vi "LED_Perform Measurements.vi"(8 "error in":errorcluster, 9 "Voltage Values":dbl[](array[numeric]), 11 "Measurement Config_In":T1={"Load channel name"="", "Load out"="", "Source out"="", "Source channel name"="", "Source sequence name"="", "Voltage values"=[], "Voltage values-CV"=[], "Voltage values-LED"=[], "Output Resistance-LED"=[], "Source terminal name"="", "Measure terminal name"="", "Load Voltage-out"=[], "Load Current - out"=[], "Source Voltage-out"=[], "Source Current - out"=[], "LED Mode Start?"=FALSE, "LED Mode Completed?"=FALSE, "CalculateRd"=0.0, "Set LED Current Limit?"=FALSE, "OutputVoltageOffset"=0.0, "measurement results"={"Status"="Empty", "Source voltages"=[0.0], "Load voltages"=[0.0], "Source current"=[0.0], "Load current"=[0.0]}}) -> (0 "error Out":errorcluster, 1 "Measurement Data":T3, 3 "Measurement Config_Out":T1={"Load channel name"="", "Load out"="", "Source out"="", "Source channel name"="", "Source sequence name"="", "Voltage values"=[], "Voltage values-CV"=[], "Voltage values-LED"=[], "Output Resistance-LED"=[], "Source terminal name"="", "Measure terminal name"="", "Load Voltage-out"=[], "Load Current - out"=[], "Source Voltage-out"=[], "Source Current - out"=[], "LED Mode Start?"=FALSE, "LED Mode Completed?"=FALSE, "CalculateRd"=0.0, "Set LED Current Limit?"=FALSE, "OutputVoltageOffset"=0.0, "measurement results"={"Status"="Empty", "Source voltages"=[0.0], "Load voltages"=[0.0], "Source current"=[0.0], "Load current"=[0.0]}})   [LabVIEW 2021, in "start-up.lvlib"]
doc: "This VI captures the Measurement data from Source and Load, for the Input Voltage."
uses:
  start-up.lvlib
  Controls/LEDStartup_Data.ctl
  Measurement Results.ctl
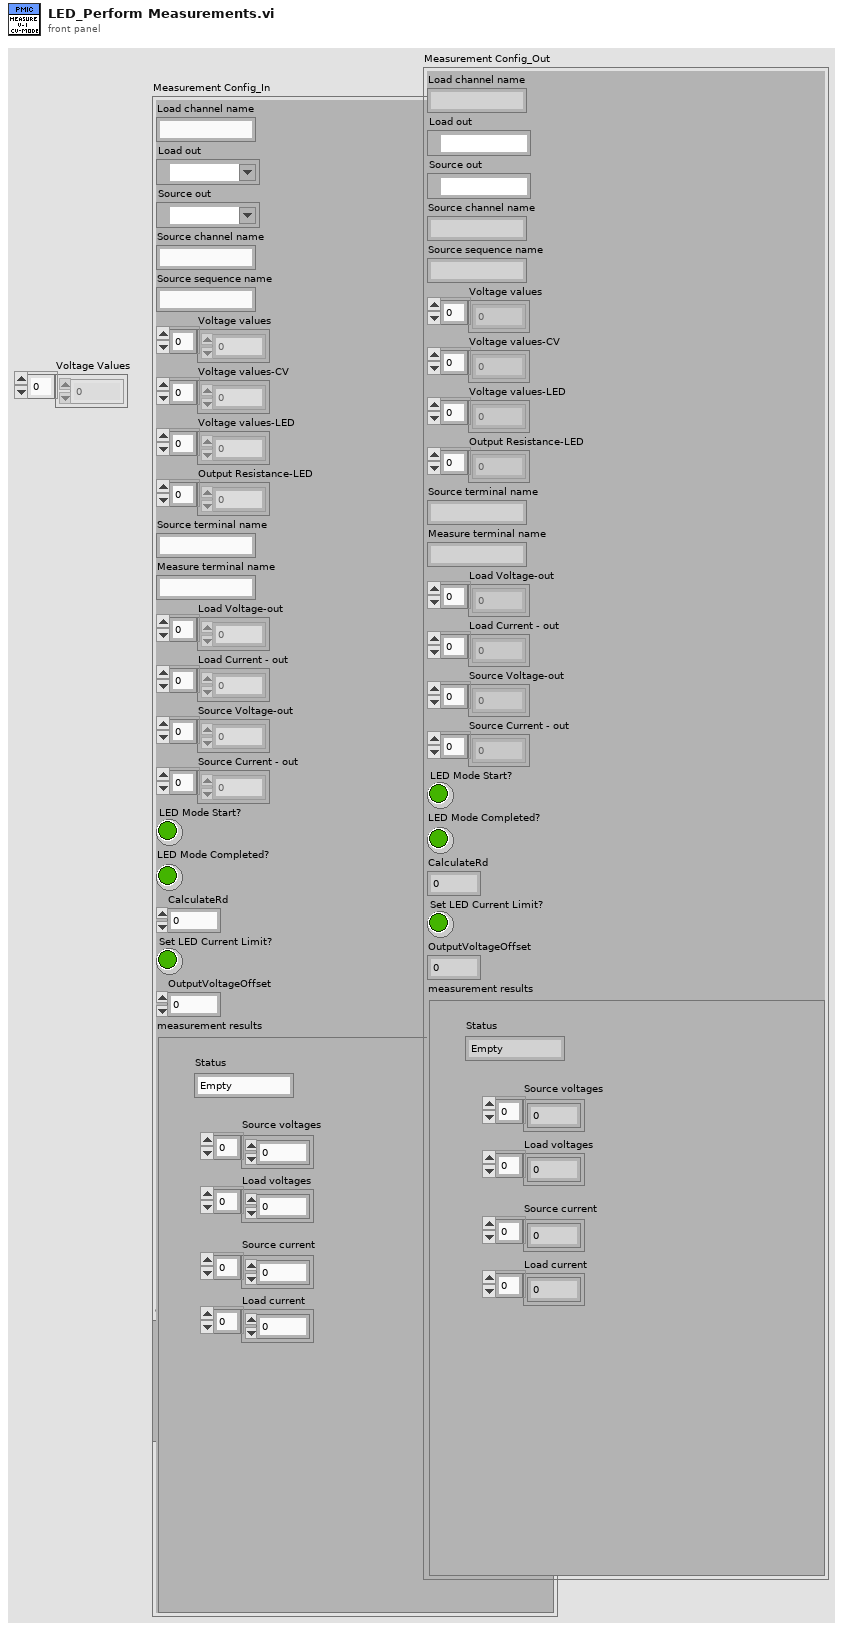
[diagram p1: front panel]
types:
  T1 = typedef "start-up.lvlib/LEDStartup_Data.ctl" = cluster{"Load channel name":string, "Load out":refnum<k15>, "Source out":refnum<k15>, "Source channel name":string, "Source sequence name":string, "Voltage values":dbl[], "Voltage values-CV":dbl[], "Voltage values-LED":dbl[], "Output Resistance-LED":dbl[], "Source terminal name":string, "Measure terminal name":string, "Load Voltage-out":dbl[], "Load Current - out":dbl[], "Source Voltage-out":dbl[], "Source Current - out":dbl[], "LED Mode Start?":bool, "LED Mode Completed?":bool, "CalculateRd":dbl, "Set LED Current Limit?":bool, "OutputVoltageOffset":dbl, "measurement results":T2}
  T2 = typedef "start-up.lvlib/Measurement Results.ctl" = cluster{"Status":string, "Source voltages":dbl[], "Load voltages":dbl[], "Source current":dbl[], "Load current":dbl[]}
  T3 = cluster{"Source Voltage":dbl[], "Source Current":dbl[], "Load Voltage":dbl[], "Load Current":dbl[]}
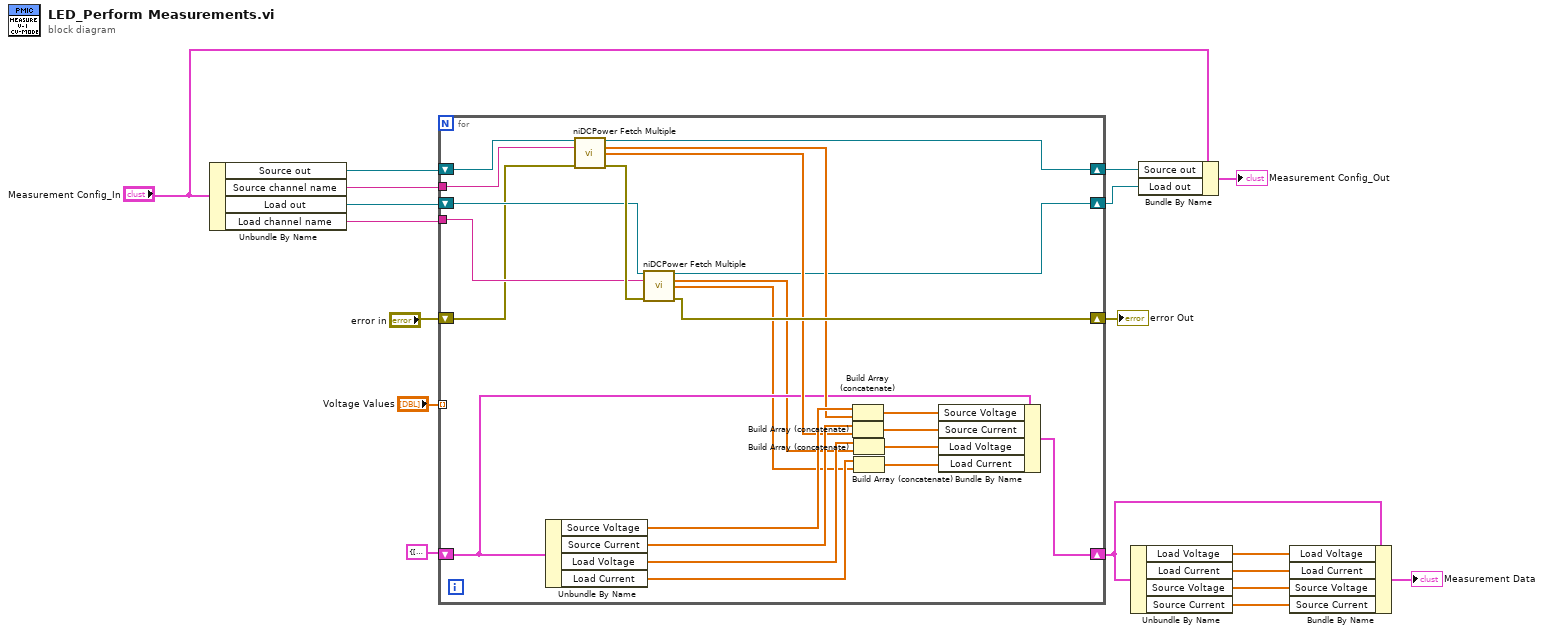
[diagram p0: block diagram]
diagram:
  n1 = Unbundle By Name("Measurement Config_In") -> ("Source out"=w18:refnum<k15>, "Source channel name"=w16:string, "Load out"=w17:refnum<k15>, "Load channel name"=w15:string)
  n2 = for {
    tunnel: w16 -> [w39]
    tunnel: w15 -> [w38]
    shift-right: [w37] -> w14
    shift-left: "error in" -> [w25]
    shift-right: [w26] -> w9
    shift-left: T3 {"Source Voltage"=[], "Source Current"=[], "Load Voltage"=[], "Load Current"=[]} -> [w31]
    tunnel: "Voltage Values" -> [_] mode=indexing
    shift-right: [w24] -> w7
    shift-left: w18 -> [w40]
    shift-right: [w23] -> w6
    shift-left: w17 -> [w36]
    n3 = Unbundle By Name(w31) -> ("Source Voltage"=w35:dbl[], "Source Current"=w33:dbl[], "Load Voltage"=w22:dbl[], "Load Current"=w20:dbl[])
    n4 = call <instrlib>:"niDCPower Fetch Multiple.vi"("instrument handle"=w40, "channel name"=w39, "error in (no error)"=w25) -> ("instrument handle out"=w24:refnum<k15>, "voltage measurements"=w34:dbl[], "current measurements"=w32:dbl[], "error out"=w41:errorcluster)  [unwired: 2 in, 7 out]
    n5 = call <instrlib>:"niDCPower Fetch Multiple.vi"("instrument handle"=w36, "channel name"=w38, "error in (no error)"=w41) -> ("instrument handle out"=w23:refnum<k15>, "voltage measurements"=w21:dbl[], "current measurements"=w19:dbl[], "error out"=w37:errorcluster)  [unwired: 2 in, 7 out]
    n6 = Build Array (concatenate)(w35, w34) -> (w30:dbl[])
    n7 = Build Array (concatenate)(w33, w32) -> (w29:dbl[])
    n8 = Build Array (concatenate)(w22, w21) -> (w28:dbl[])
    n9 = Build Array (concatenate)(w20, w19) -> (w27:dbl[])
    n10 = Bundle By Name(cluster=w31, "Source Voltage"=w30, "Source Current"=w29, "Load Voltage"=w28, "Load Current"=w27) -> (w26:T3)
  }
  "error Out" <- w14
  n11 = Unbundle By Name(w9) -> ("Load Voltage"=w11:dbl[], "Load Current"=w10:dbl[], "Source Voltage"=w5:dbl[], "Source Current"=w4:dbl[])
  n12 = Bundle By Name(cluster="Measurement Config_In", "Source out"=w7, "Load out"=w6) -> (→"Measurement Config_Out":T1)
  n13 = Bundle By Name(cluster=w9, "Load Voltage"=w11, "Load Current"=w10, "Source Voltage"=w5, "Source Current"=w4) -> (→"Measurement Data":T3)
